vi "Digital Debounce Filter.vi"(7 "Cycles to Filter":u64=5, 8 "Previous Count":u64, 10 "Previous Input Signal":bool, 11 "Input Signal":bool) -> (0 "Count":u64, 3 "Output Filtered Signal":bool)   [LabVIEW 2019, in "Control Addon Engine.lvlib"]
uses:
  Control Addon Engine.lvlib
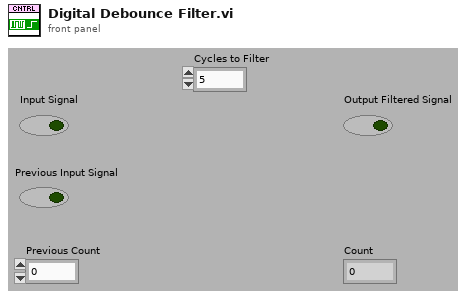
[diagram p1: front panel]
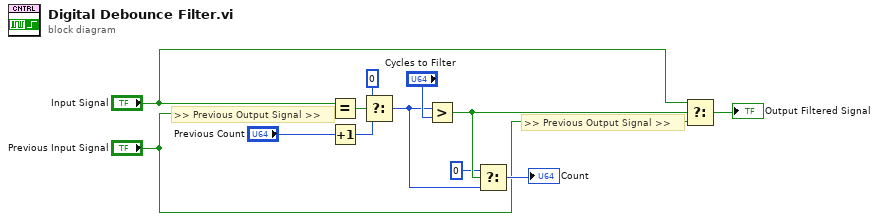
[diagram p0: block diagram]
diagram:
  # ">> Previous Output Signal >>"
  # ">> Previous Output Signal >>"
  n1 = Equal?(x="Input Signal", y="Previous Input Signal") -> (x = y?=w9:bool)
  n2 = Increment(x="Previous Count") -> (x+1=w7:u64)
  n3 = Select(t=u64 0 ("f"), s=w9, f=w7) -> (s? t:f=w4:u64)
  n4 = Greater?(x=w4, y="Cycles to Filter") -> (0:w6:bool)
  n5 = Select(t=u64 0, s=w6, f=w4) -> (s? t:f=→"Count":u64)
  n6 = Select(t="Input Signal", s=w6, f="Previous Input Signal") -> (s? t:f=→"Output Filtered Signal":bool)
